vi "Error Handler - Message Handling Loop.vi"(8 "error in (no error)":errorcluster, 10 "Ignore Errors (Runtime)":i32[](array[numeric]), 11 "Message Queue":refnum<queue>) -> (0 "dup error in":errorcluster, 3 "dup Message Queue":refnum<queue>)   [LabVIEW 2016]
doc: "Process an error that occurred in the Message Handling Loop, either by ignoring it, or generating an \"Error\" message."
uses:
  Message Queue/Message Cluster.ctl
  Message Queue/Message Queue.lvlib
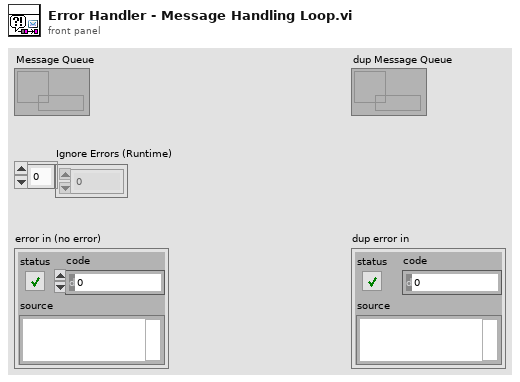
[diagram p1: front panel]
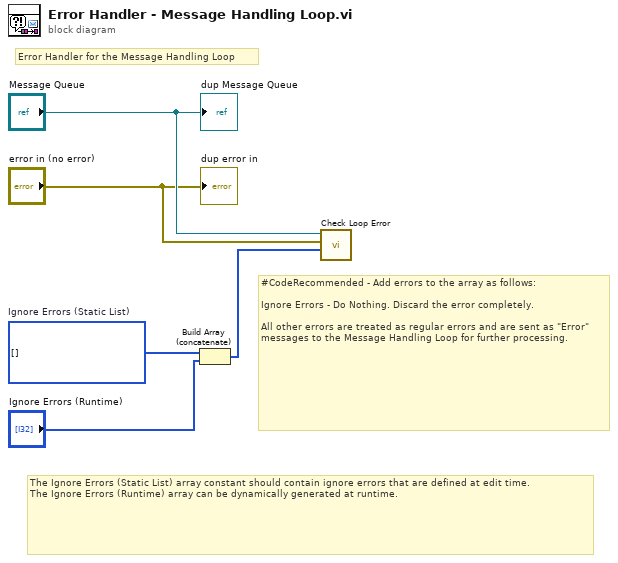
[diagram p0: block diagram]
diagram:
  w3 = i32[] []  # Ignore Errors (Static List)
  # "The Ignore Errors (Static List) array constant should contain ignore errors that are defined at edit time.\nThe Ignore Errors (Runtime) array can be dynamically generated at runtime."
  # "#CodeRecommended - Add errors to the array as follows:\n\nIgnore Errors - Do Nothing. Discard the error completely.\n\nAll other errors are treated as regular errors and are sent as \"Error\" messages to the Message Handling Loop for further processing."
  # "Error Handler for the Message Handling Loop"
  n1 = Build Array (concatenate)(w3, "Ignore Errors (Runtime)") -> (w1:i32[])
  n2 = call "Check Loop Error.vi"("Ignore Errors"=w1, "error to process"="error in (no error)", "Message Queue"="Message Queue") -> ()  [unwired: 7 in, 2 out]
  "dup Message Queue" <- "Message Queue"
  "dup error in" <- "error in (no error)"
